vi "FPGA_MAIN.vi"() -> ()   [LabVIEW 2019]
uses:
  <vilib>/LabVIEW Targets/FPGA/RIO/nicrio_985x_controls.llb/CAN_IO_Frame Cluster.ctl
  <vilib>/LabVIEW Targets/FPGA/RIO/nicrio_985x_controls.llb/CAN_IO_Frame Type.ctl
  <vilib>/rvi/Emulation/niFpgaGetClockAttributes.vi
  <vilib>/rvi/Emulation/niFpgaSctlEmulationGetInTimedLoop.vi
  <vilib>/rvi/Emulation/niFpgaEmulationReportErrorSimple.vi
  <vilib>/rvi/eio/common/nirviEmuTemplateMethod_errors.vi
  <vilib>/rvi/Emulation/niFpgaCriticalErrorInLSC.vi
  <vilib>/eio/EIONode/EIONode.xnode
panel:
  out "Save_que_indicator":bool
  in  "Save_que":bool
  out "IMUS":sgl[](array[numeric])
  out "Mod1/CAN0":T1={"timestamp high"=0, "timestamp low"=0, "identifier"=0, "type"=enum."Data Frame", "info A"=0, "info B"=0, "data length"=0, "data"=[0, 0, 0, 0, 0, 0, 0, 0]} {"identifier" format="%x"; "timestamp high" format="%08x"; "timestamp low" format="%08x"; "data" format="%.0x"}
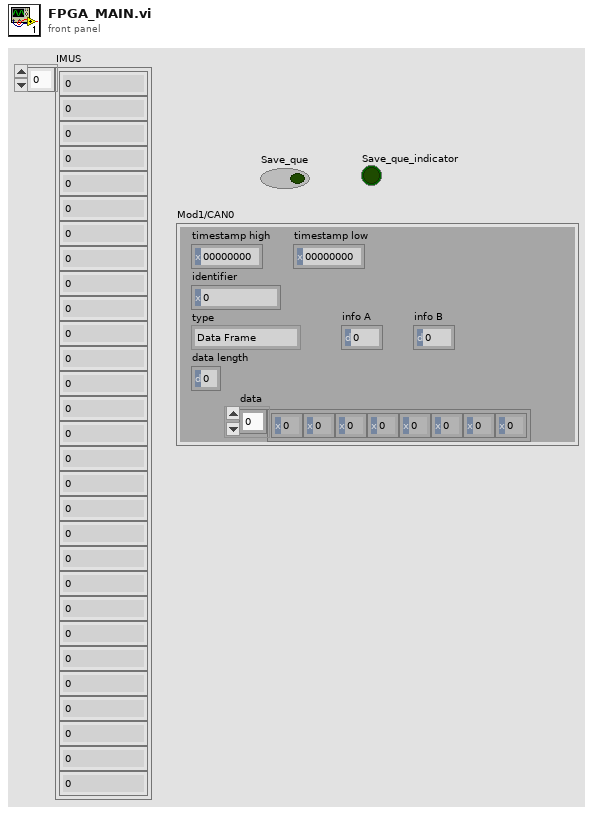
[diagram p1: front panel]
types:
  T1 = typedef "CAN_IO_Frame Cluster.ctl" = cluster{"timestamp high":u32, "timestamp low":u32, "identifier":u32, "type":T2, "info A":u8, "info B":u8, "data length":u8, "data":u8[]}
  T2 = typedef "CAN_IO_Frame Type.ctl" = enum8{"Data Frame", "Remote Frame", "(reserved)", "(reserved) ", "(reserved)  ", "(reserved)   ", "Bus Error", "Transceiver Fault"}
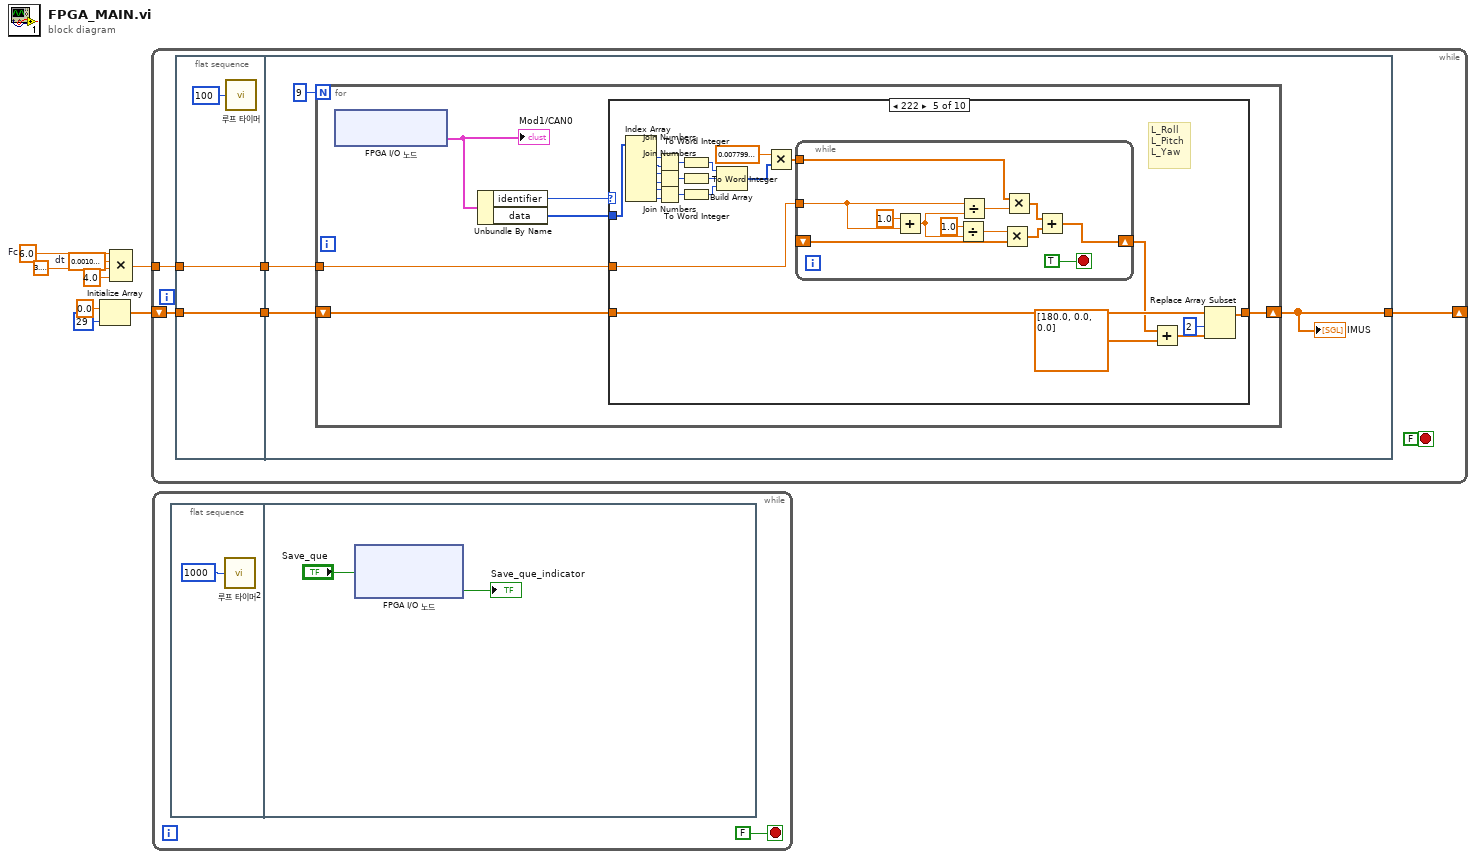
[diagram p0: block diagram]
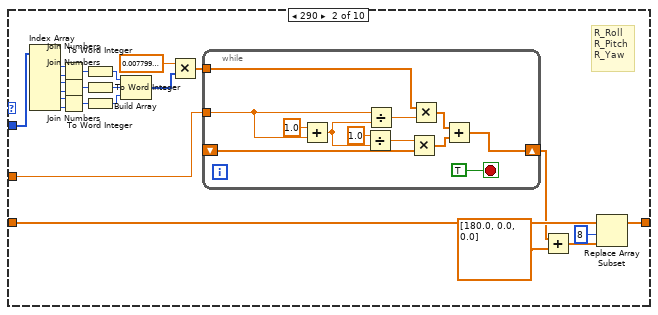
[diagram p3: hidden frame]
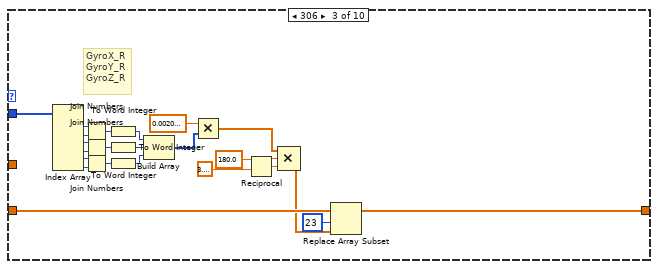
[diagram p4: hidden frame]
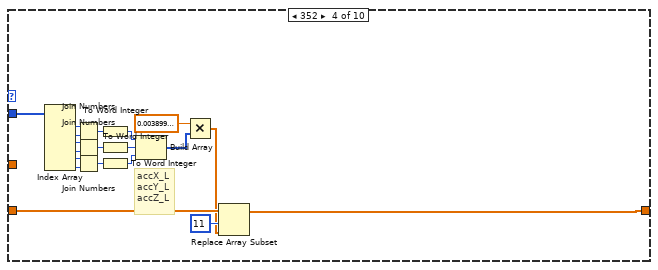
[diagram p5: hidden frame]
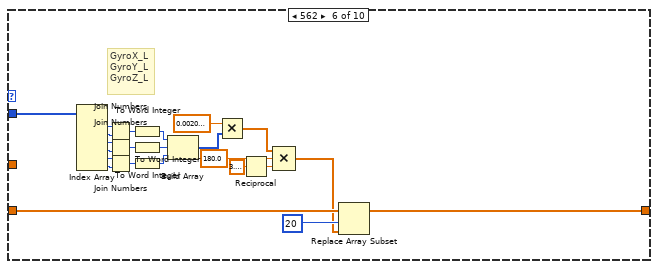
[diagram p6: hidden frame]
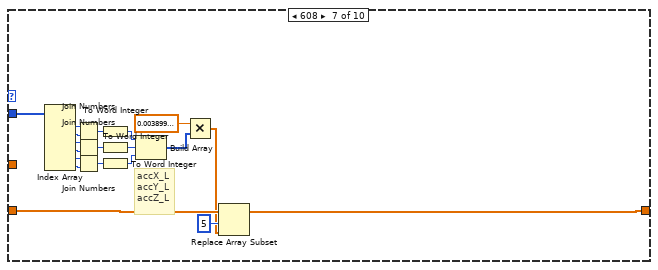
[diagram p7: hidden frame]
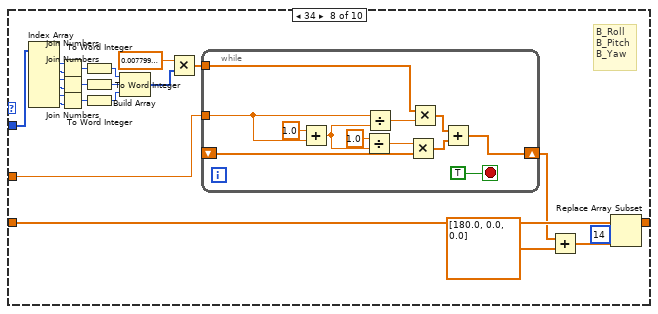
[diagram p8: hidden frame]
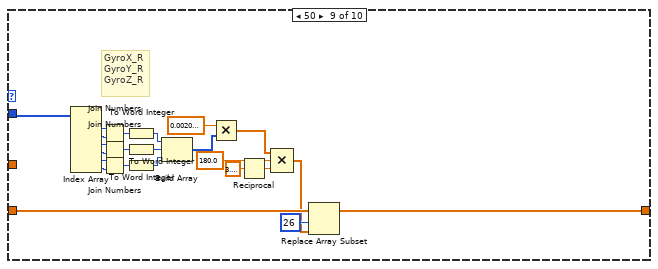
[diagram p9: hidden frame]
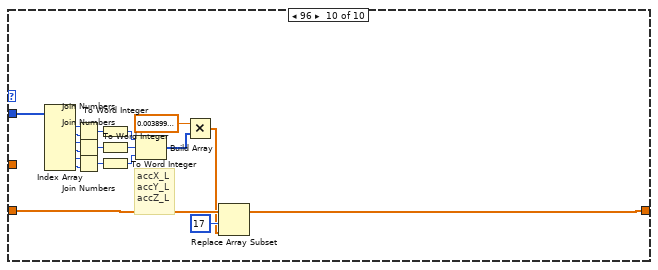
[diagram p10: hidden frame]
diagram:
  w4 = sgl 0.001  # dt
  w5 = sgl 6.0  # Fc
  n1 = Initialize Array(sgl 0.0 ("timeout (0 s)"), 29 ("차원 크기")) -> (w6:sgl[])
  n2 = Compound Arithmetic op=MULTIPLY ("복합 연산")(w5, w4, sgl 3.1415927, sgl 4.0 ("값")) -> (w1:sgl)
  n3 = while {
    shift-right: [w13] -> _
    shift-left: w6 -> [w12]
    tunnel: w1 -> [w9]
    stop <- FALSE stop-if-true
    n4 = flat-sequence {
      tunnel: w12 -> [w16]
      tunnel: [w16] -> w11
      tunnel: [w15] -> w10
      tunnel: w9 -> [w15]
      tunnel: [w21] -> w13
      tunnel: w11 -> [w20]
      tunnel: w10 -> [w19]
      frame #0 {
        n5 = call "루프 타이머"("Count(uSec)"=u32 100 ("Count(mSec)")) -> ()  [unwired: 1 out]
      }
      frame #1 {
        n6 = for {
          N: 9 -> [_]
          tunnel: w19 -> [w22]
          shift-right: [w24] -> w21
          shift-left: w20 -> [w23]
          n7 = xnode "FPGA I/O 노드"() -> ("Mod1/CAN0"=w25:T1)  [unwired: 1 in, 1 out]
          "Mod1/CAN0" <- w25
          n8 = Unbundle By Name(w25) -> ("identifier"=w27:u32, "data"=w26:u8[])
          n9 = case shown="222" w27 {
            tunnel: w26 -> [_ w51 w71 w99 w128 w148 w176 w205 w225 w253]
            tunnel: w23 -> [w28 w49 w70 w98 w109 w147 w175 w203 w224 w252]
            tunnel: [w28 w29 w69 w96 w106 w146 w173 w183 w223 w250] -> w24
            tunnel: w22 -> [_ w50 _ _ w127 _ _ w204 _ _]
            frame 0, Default {
            }
            frame 290 {
              # "R_Roll\nR_Pitch\nR_Yaw"
              n10 = Index Array(array=w51) -> (element #1=w43:u8, element #2=w44:u8, element #3=w45:u8, element #4=w46:u8, element #5=w47:u8, element #6=w48:u8)  [unwired: 6 in]
              n11 = Join Numbers(hi=w43, lo=w44) -> ((hi.lo)=w40:u16)
              n12 = Join Numbers(hi=w45, lo=w46) -> ((hi.lo)=w38:u16)
              n13 = Join Numbers(hi=w47, lo=w48) -> ((hi.lo)=w39:u16)
              n14 = To Word Integer(number=w40) -> (16bit integer=w36:i16)
              n15 = To Word Integer(number=w38) -> (16bit integer=w35:i16)
              n16 = To Word Integer(number=w39) -> (16bit integer=w34:i16)
              n17 = Build Array(w36, w35, w34) -> (w33:i16[])
              n18 = Multiply ("곱하기")(x=sgl 0.0078, y=w33) -> (x*y=w31:sgl[])
              n19 = while {
                tunnel: w50 -> [w52]
                tunnel: w31 -> [w55]
                shift-right: [w54] -> w30
                shift-left: _ -> [w53]
                stop <- TRUE stop-if-true
                n20 = Add(x=sgl 1.0, y=w52) -> (x+y=w59:sgl)
                n21 = Divide(x=sgl 1.0, y=w59) -> (x/y=w56:sgl)
                n22 = Divide ("나누기")(x=w52, y=w59) -> (x/y=w62:sgl)
                n23 = Multiply(x=w56, y=w53) -> (x*y=w57:sgl[])
                n24 = Multiply(x=w55, y=w62) -> (x*y=w58:sgl[])
                n25 = Add(x=w58, y=w57) -> (x+y=w54:sgl[])
              }
              n26 = Add(x=w30, y=sgl[] [180.0, 0.0, 0.0]) -> (x+y=w41:sgl[])
              n27 = Replace Array Subset(array=w49, new element=w41, index=8 ("인덱스")) -> (w29:sgl[])
            }
            frame 306 {
              # "GyroX_R\nGyroY_R\nGyroZ_R"
              n28 = Index Array(array=w71) -> (element #1=w81:u8, element #2=w82:u8, element #3=w83:u8, element #4=w84:u8, element #5=w85:u8, element #6=w86:u8)  [unwired: 6 in]
              n29 = Join Numbers(hi=w81, lo=w82) -> ((hi.lo)=w79:u16)
              n30 = Join Numbers(hi=w83, lo=w84) -> ((hi.lo)=w77:u16)
              n31 = Join Numbers(hi=w85, lo=w86) -> ((hi.lo)=w78:u16)
              n32 = To Word Integer(number=w79) -> (16bit integer=w75:i16)
              n33 = To Word Integer(number=w77) -> (16bit integer=w74:i16)
              n34 = To Word Integer(number=w78) -> (16bit integer=w73:i16)
              n35 = Build Array(w75, w74, w73) -> (w72:i16[])
              n36 = Multiply ("곱하기")(x=sgl 0.002, y=w72) -> (x*y=w68:sgl[])
              n37 = Reciprocal(x=sgl 3.1415927) -> (1/x=w67:sgl)
              n38 = Compound Arithmetic op=MULTIPLY(w68, sgl 180.0 ("값"), w67) -> (w66:sgl[])
              n39 = Replace Array Subset(array=w70, new element=w66, index=23 ("인덱스")) -> (w69:sgl[])
            }
            frame 352 {
              # "accX_L\naccY_L\naccZ_L"
              n40 = Index Array(array=w99) -> (element #1=w100:u8, element #2=w101:u8, element #3=w102:u8, element #4=w103:u8, element #5=w104:u8, element #6=w105:u8)  [unwired: 6 in]
              n41 = Join Numbers(hi=w100, lo=w101) -> ((hi.lo)=w95:u16)
              n42 = Join Numbers(hi=w102, lo=w103) -> ((hi.lo)=w93:u16)
              n43 = Join Numbers(hi=w104, lo=w105) -> ((hi.lo)=w94:u16)
              n44 = To Word Integer(number=w95) -> (16bit integer=w91:i16)
              n45 = To Word Integer(number=w93) -> (16bit integer=w90:i16)
              n46 = To Word Integer(number=w94) -> (16bit integer=w89:i16)
              n47 = Build Array(w91, w90, w89) -> (w88:i16[])
              n48 = Multiply ("곱하기")(x=sgl 0.0039, y=w88) -> (x*y=w87:sgl[])
              n49 = Replace Array Subset(array=w98, new element=w87, index=11 ("인덱스")) -> (w96:sgl[])
            }
            frame 546 {
              # "L_Roll\nL_Pitch\nL_Yaw"
              n50 = Index Array(array=w128) -> (element #1=w121:u8, element #2=w122:u8, element #3=w123:u8, element #4=w124:u8, element #5=w125:u8, element #6=w126:u8)  [unwired: 6 in]
              n51 = Join Numbers(hi=w121, lo=w122) -> ((hi.lo)=w118:u16)
              n52 = Join Numbers(hi=w123, lo=w124) -> ((hi.lo)=w116:u16)
              n53 = Join Numbers(hi=w125, lo=w126) -> ((hi.lo)=w117:u16)
              n54 = To Word Integer(number=w118) -> (16bit integer=w114:i16)
              n55 = To Word Integer(number=w116) -> (16bit integer=w113:i16)
              n56 = To Word Integer(number=w117) -> (16bit integer=w112:i16)
              n57 = Build Array(w114, w113, w112) -> (w111:i16[])
              n58 = Multiply ("곱하기")(x=sgl 0.0078, y=w111) -> (x*y=w107:sgl[])
              n59 = while {
                tunnel: w127 -> [w129]
                tunnel: w107 -> [w132]
                shift-right: [w131] -> w108
                shift-left: _ -> [w130]
                stop <- TRUE stop-if-true
                n60 = Add(x=sgl 1.0, y=w129) -> (x+y=w136:sgl)
                n61 = Divide(x=sgl 1.0, y=w136) -> (x/y=w133:sgl)
                n62 = Divide ("나누기")(x=w129, y=w136) -> (x/y=w139:sgl)
                n63 = Multiply(x=w133, y=w130) -> (x*y=w134:sgl[])
                n64 = Multiply(x=w132, y=w139) -> (x*y=w135:sgl[])
                n65 = Add(x=w135, y=w134) -> (x+y=w131:sgl[])
              }
              n66 = Add(x=w108, y=sgl[] [180.0, 0.0, 0.0]) -> (x+y=w119:sgl[])
              n67 = Replace Array Subset(array=w109, new element=w119, index=2 ("인덱스")) -> (w106:sgl[])
            }
            frame 562 {
              # "GyroX_L\nGyroY_L\nGyroZ_L"
              n68 = Index Array(array=w148) -> (element #1=w156:u8, element #2=w155:u8, element #3=w154:u8, element #4=w153:u8, element #5=w152:u8, element #6=w151:u8)  [unwired: 6 in]
              n69 = Join Numbers(hi=w156, lo=w155) -> ((hi.lo)=w157:u16)
              n70 = Join Numbers(hi=w154, lo=w153) -> ((hi.lo)=w159:u16)
              n71 = Join Numbers(hi=w152, lo=w151) -> ((hi.lo)=w158:u16)
              n72 = To Word Integer(number=w157) -> (16bit integer=w160:i16)
              n73 = To Word Integer(number=w159) -> (16bit integer=w161:i16)
              n74 = To Word Integer(number=w158) -> (16bit integer=w162:i16)
              n75 = Build Array(w160, w161, w162) -> (w163:i16[])
              n76 = Multiply ("곱하기")(x=sgl 0.002, y=w163) -> (x*y=w144:sgl[])
              n77 = Reciprocal(x=sgl 3.1415927) -> (1/x=w145:sgl)
              n78 = Compound Arithmetic op=MULTIPLY(w144, sgl 180.0 ("값"), w145) -> (w143:sgl[])
              n79 = Replace Array Subset(array=w147, new element=w143, index=20 ("인덱스")) -> (w146:sgl[])
            }
            frame 608 {
              # "accX_L\naccY_L\naccZ_L"
              n80 = Index Array(array=w176) -> (element #1=w177:u8, element #2=w178:u8, element #3=w179:u8, element #4=w180:u8, element #5=w181:u8, element #6=w182:u8)  [unwired: 6 in]
              n81 = Join Numbers(hi=w177, lo=w178) -> ((hi.lo)=w172:u16)
              n82 = Join Numbers(hi=w179, lo=w180) -> ((hi.lo)=w170:u16)
              n83 = Join Numbers(hi=w181, lo=w182) -> ((hi.lo)=w171:u16)
              n84 = To Word Integer(number=w172) -> (16bit integer=w168:i16)
              n85 = To Word Integer(number=w170) -> (16bit integer=w167:i16)
              n86 = To Word Integer(number=w171) -> (16bit integer=w166:i16)
              n87 = Build Array(w168, w167, w166) -> (w165:i16[])
              n88 = Multiply ("곱하기")(x=sgl 0.0039, y=w165) -> (x*y=w164:sgl[])
              n89 = Replace Array Subset(array=w175, new element=w164, index=5 ("인덱스")) -> (w173:sgl[])
            }
            frame 34 {
              # "B_Roll\nB_Pitch\nB_Yaw"
              n90 = Index Array(array=w205) -> (element #1=w197:u8, element #2=w198:u8, element #3=w199:u8, element #4=w200:u8, element #5=w201:u8, element #6=w202:u8)  [unwired: 6 in]
              n91 = Join Numbers(hi=w197, lo=w198) -> ((hi.lo)=w194:u16)
              n92 = Join Numbers(hi=w199, lo=w200) -> ((hi.lo)=w192:u16)
              n93 = Join Numbers(hi=w201, lo=w202) -> ((hi.lo)=w193:u16)
              n94 = To Word Integer(number=w194) -> (16bit integer=w190:i16)
              n95 = To Word Integer(number=w192) -> (16bit integer=w189:i16)
              n96 = To Word Integer(number=w193) -> (16bit integer=w188:i16)
              n97 = Build Array(w190, w189, w188) -> (w187:i16[])
              n98 = Multiply ("곱하기")(x=sgl 0.0078, y=w187) -> (x*y=w185:sgl[])
              n99 = while {
                tunnel: w204 -> [w206]
                tunnel: w185 -> [w209]
                shift-right: [w208] -> w184
                shift-left: _ -> [w207]
                stop <- TRUE stop-if-true
                n100 = Add(x=sgl 1.0, y=w206) -> (x+y=w213:sgl)
                n101 = Divide(x=sgl 1.0, y=w213) -> (x/y=w210:sgl)
                n102 = Divide ("나누기")(x=w206, y=w213) -> (x/y=w216:sgl)
                n103 = Multiply(x=w210, y=w207) -> (x*y=w211:sgl[])
                n104 = Multiply(x=w209, y=w216) -> (x*y=w212:sgl[])
                n105 = Add(x=w212, y=w211) -> (x+y=w208:sgl[])
              }
              n106 = Add(x=w184, y=sgl[] [180.0, 0.0, 0.0]) -> (x+y=w195:sgl[])
              n107 = Replace Array Subset(array=w203, new element=w195, index=14 ("인덱스")) -> (w183:sgl[])
            }
            frame 50 {
              # "GyroX_R\nGyroY_R\nGyroZ_R"
              n108 = Index Array(array=w225) -> (element #1=w235:u8, element #2=w236:u8, element #3=w237:u8, element #4=w238:u8, element #5=w239:u8, element #6=w240:u8)  [unwired: 6 in]
              n109 = Join Numbers(hi=w235, lo=w236) -> ((hi.lo)=w233:u16)
              n110 = Join Numbers(hi=w237, lo=w238) -> ((hi.lo)=w231:u16)
              n111 = Join Numbers(hi=w239, lo=w240) -> ((hi.lo)=w232:u16)
              n112 = To Word Integer(number=w233) -> (16bit integer=w229:i16)
              n113 = To Word Integer(number=w231) -> (16bit integer=w228:i16)
              n114 = To Word Integer(number=w232) -> (16bit integer=w227:i16)
              n115 = Build Array(w229, w228, w227) -> (w226:i16[])
              n116 = Multiply ("곱하기")(x=sgl 0.002, y=w226) -> (x*y=w221:sgl[])
              n117 = Reciprocal(x=sgl 3.1415927) -> (1/x=w222:sgl)
              n118 = Compound Arithmetic op=MULTIPLY(w221, sgl 180.0 ("값"), w222) -> (w220:sgl[])
              n119 = Replace Array Subset(array=w224, new element=w220, index=26 ("인덱스")) -> (w223:sgl[])
            }
            frame 96 {
              # "accX_L\naccY_L\naccZ_L"
              n120 = Index Array(array=w253) -> (element #1=w254:u8, element #2=w255:u8, element #3=w256:u8, element #4=w257:u8, element #5=w258:u8, element #6=w259:u8)  [unwired: 6 in]
              n121 = Join Numbers(hi=w254, lo=w255) -> ((hi.lo)=w249:u16)
              n122 = Join Numbers(hi=w256, lo=w257) -> ((hi.lo)=w247:u16)
              n123 = Join Numbers(hi=w258, lo=w259) -> ((hi.lo)=w248:u16)
              n124 = To Word Integer(number=w249) -> (16bit integer=w245:i16)
              n125 = To Word Integer(number=w247) -> (16bit integer=w244:i16)
              n126 = To Word Integer(number=w248) -> (16bit integer=w243:i16)
              n127 = Build Array(w245, w244, w243) -> (w242:i16[])
              n128 = Multiply ("곱하기")(x=sgl 0.0039, y=w242) -> (x*y=w241:sgl[])
              n129 = Replace Array Subset(array=w252, new element=w241, index=17 ("인덱스")) -> (w250:sgl[])
            }
          }
        }
        "IMUS" <- w21
      }
    }
  }
  n130 = while {
    stop <- FALSE stop-if-true
    n131 = flat-sequence {
      frame #0 {
        n132 = call "루프 타이머2"("Count(uSec)"=u32 1000 ("Count(mSec)")) -> ()  [unwired: 1 out]
      }
      frame #1 {
        n133 = xnode "FPGA I/O 노드"("Mod3/DIO0"="Save_que") -> ("Mod3/DIO0"=→"Save_que_indicator":bool)  [unwired: 2 in, 2 out]
      }
    }
  }
